vi "Least Common Multiple (LCM)-scalar input.vi"(8 "error in (no error)":errorcluster, 10 "y":i32, 11 "x":i32) -> (0 "error out":errorcluster, 3 "Least Common Multiple (LCM)":i32)   [LabVIEW 2021, in "Numeric Utilities.lvlib"]
uses:
  Numeric Utilities.lvlib
  Factors cluster.ctl
panel:
  out "x factors list":T1[](array[typedef])
  out "y factors list":T1[](array[typedef])
  out "no. of distinct prime factors (y)":i32
  out "no. of distinct prime factors (x)":i32
  # "Development\ncontrols/indicators useful for development and testing, but which are not outputs of the VI"
  # "Input\nInputs to the VI"
  # "Output\nOutputs of the VI"
  # "Description\n\nBlank VI with error handling case. \n\nSummarize the use of this VI in this space."
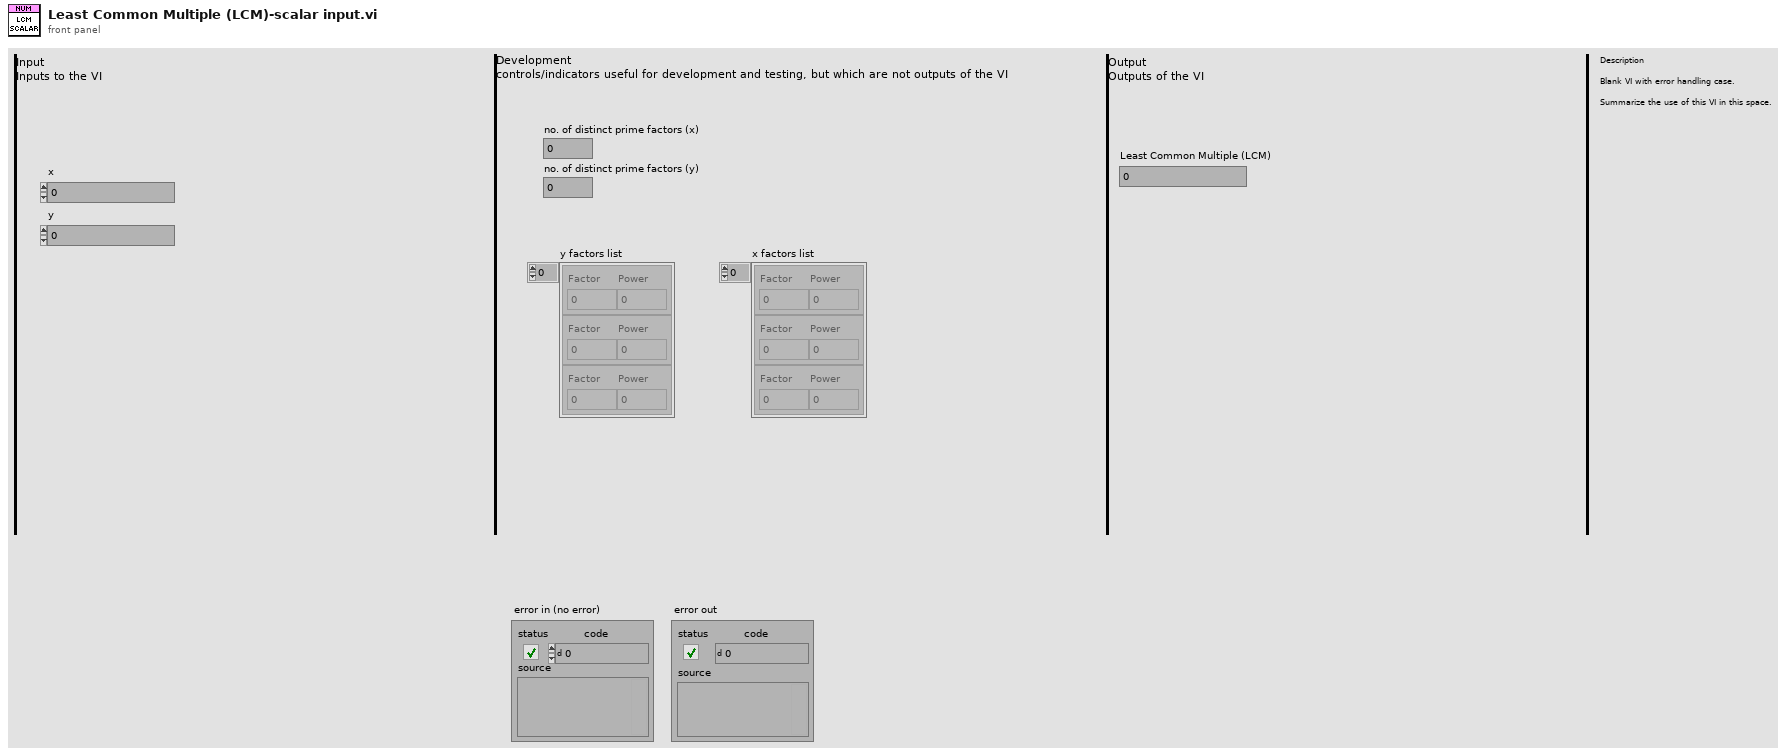
[diagram p1: front panel]
types:
  T1 = typedef "Numeric Utilities.lvlib/Factors cluster.ctl" = cluster{"Factor":i32, "Power":i32}
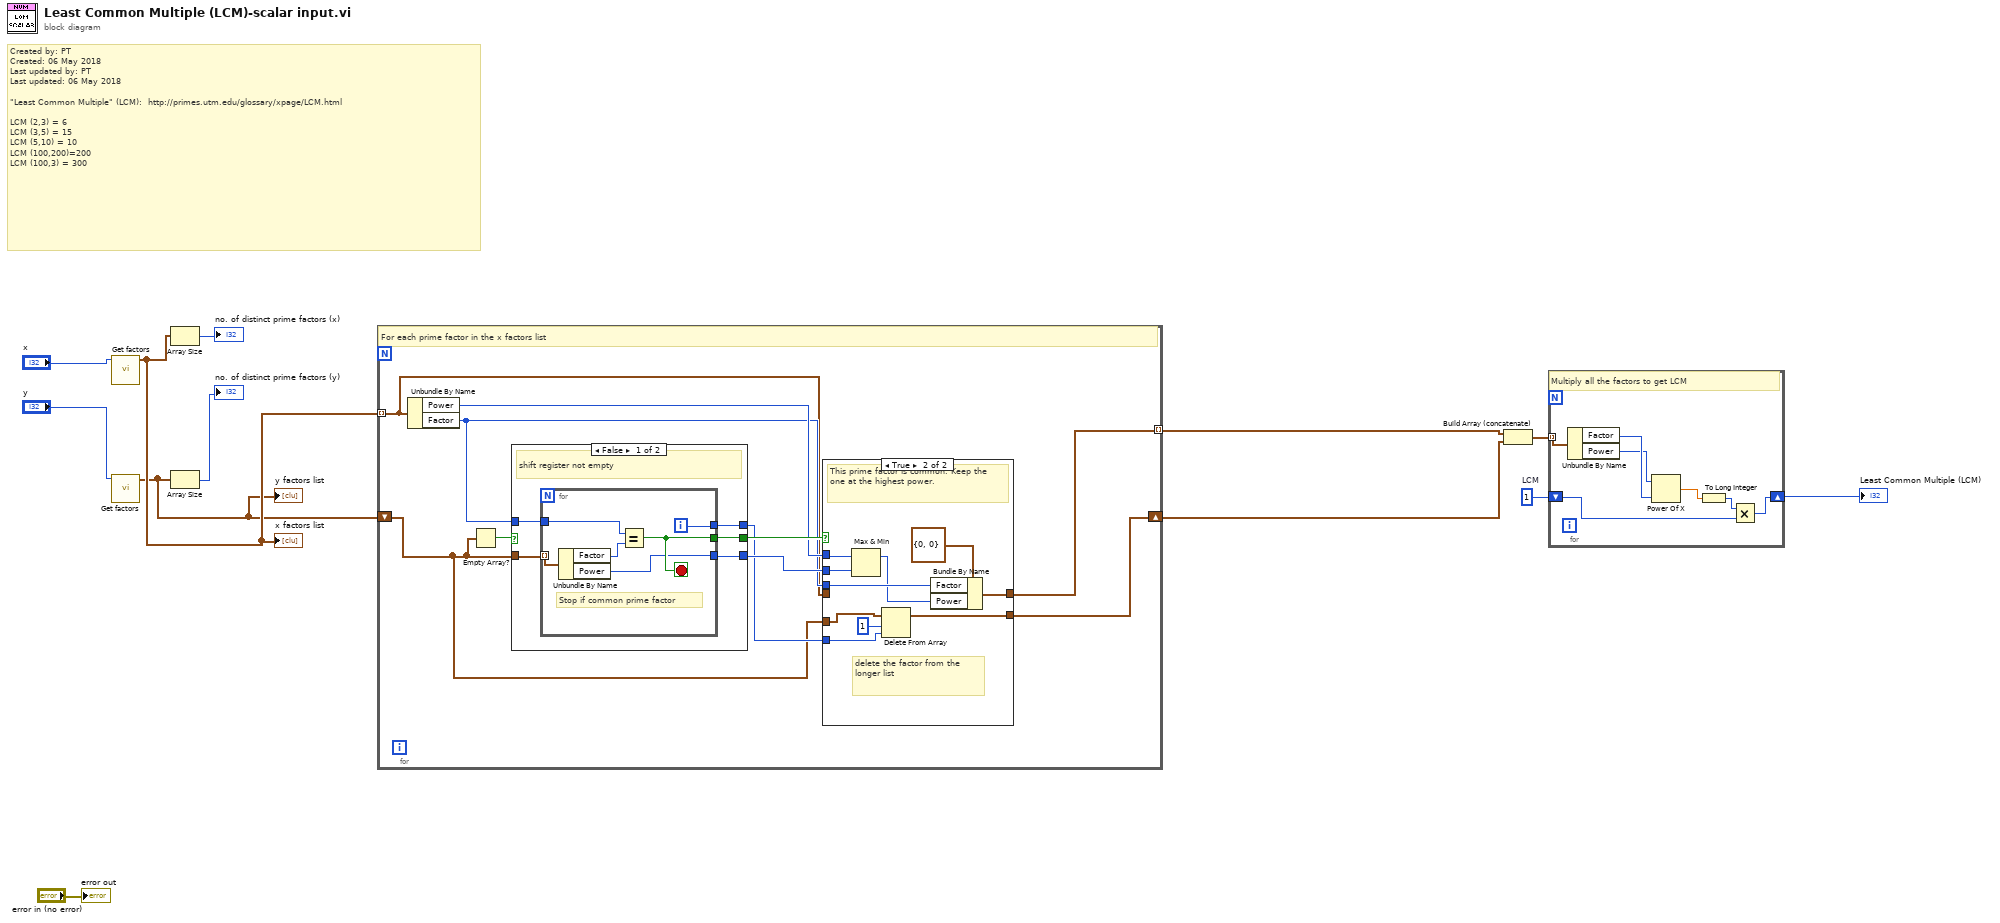
[diagram p0: block diagram]
diagram:
  w2 = 1  # LCM
  # "Created by: PT\nCreated: 06 May 2018\nLast updated by: PT\nLast updated: 06 May 2018\n\n\"Least Common Multiple\" (LCM):  http://primes.utm.edu/glossary/xpage/LCM.html\n\nLCM (2,3) = 6\nLCM (3,5) = 15\nLCM (5,10) = 10\nLCM (100,200)=200\nLCM (100,3) = 300"
  n1 = call "Get factors.vi"("x"="x") -> ("Factors out"=w7:T1[])  [unwired: 5 in, 5 out]
  "x factors list" <- w7
  n2 = call "Get factors.vi"("x"="y") -> ("Factors out"=w6:T1[])  [unwired: 5 in, 5 out]
  "y factors list" <- w6
  n3 = Array Size(array=w7) -> (size(s)=→"no. of distinct prime factors (x)":i32)
  n4 = Array Size(array=w6) -> (size(s)=→"no. of distinct prime factors (y)":i32)
  n5 = for {
    tunnel: w7 -> [w18] mode=indexing
    shift-right: [w16] -> w4
    shift-left: w6 -> [w15]
    tunnel: [w13] -> w5 mode=indexing
    # "For each prime factor in the x factors list"
    n6 = Unbundle By Name(w18) -> ("Power"=w21:i32, "Factor"=w19:i32)
    n7 = Empty Array?(array=w15) -> (empty?=w14:bool)
    n8 = case shown="False" w14 {
      tunnel: [w27 _] -> w22
      tunnel: [w26 _] -> w20
      tunnel: w19 -> [w25 _]
      tunnel: w15 -> [w24 _]
      tunnel: [w23 _] -> w17
      frame False {
        # "shift register not empty"
        n9 = for {
          tunnel: w24 -> [w33] mode=indexing
          tunnel: w25 -> [w32]
          tunnel: [w30] -> w23
          tunnel: [w29] -> w27
          tunnel: [w28] -> w26
          i -> [w30]
          stop <- w29 stop-if-true
          # "Stop if common prime factor"
          n10 = Unbundle By Name(w33) -> ("Factor"=w31:i32, "Power"=w28:i32)
          n11 = Equal?(x=w32, y=w31) -> (x = y?=w29:bool)
        }
      }
      frame True {
        # "shift register is empty."
      }
    }
    n12 = case shown="True" w22 {
      tunnel: w21 -> [_ w45]
      tunnel: w20 -> [_ w44]
      tunnel: w19 -> [_ w42]
      tunnel: [w35 w40] -> w13
      tunnel: w18 -> [w35 _]
      tunnel: w15 -> [w34 w39]
      tunnel: w17 -> [_ w37]
      tunnel: [w34 w36] -> w16
      frame False {
        # "This factor is found in the shorter list  only."
      }
      frame True {
        # "delete the factor from the longer list"
        # "This prime factor is common. Keep the one at the highest power."
        n13 = Max & Min(x=w45, y=w44) -> (max(x,y)=w41:i32)  [unwired: 1 out]
        n14 = Delete From Array(array=w39, length=1, index=w37) -> (array with subset deleted=w36:T1[])  [unwired: 1 out]
        n15 = Bundle By Name(cluster=T1 {"Factor"=0, "Power"=0} ("Factors cluster"), "Factor"=w42, "Power"=w41) -> (w40:T1)
      }
    }
  }
  n16 = Build Array (concatenate)(w5, w4) -> (w3:T1[])
  n17 = for {
    tunnel: w3 -> [w52] mode=indexing
    shift-right: [w46] -> w1
    shift-left: w2 -> [w47]
    # "Multiply all the factors to get LCM"
    n18 = Unbundle By Name(w52) -> ("Factor"=w51:i32, "Power"=w50:i32)
    n19 = Power Of X(1:w51, 2:w50) -> (0:w49:dbl)
    n20 = To Long Integer(number=w49) -> (32bit integer=w48:i32)
    n21 = Multiply(x=w48, y=w47) -> (x*y=w46:i32)
  }
  "Least Common Multiple (LCM)" <- w1
  "error out" <- "error in (no error)"
